vi "ST_parse_results_audit.vi"(7 "data_start_index":i32, 8 "error_in":errorcluster, 11 "results_from_PLC":u8[](array[numeric])) -> (0 "error_out":errorcluster, 3 "results_from_PLC":T1)   [LabVIEW 2020]
uses:
  ST_results_info.ctl
  results_byte_offset/res_REAL_offset.vi
  _misc/byte_array_parser/to_SGL.vi
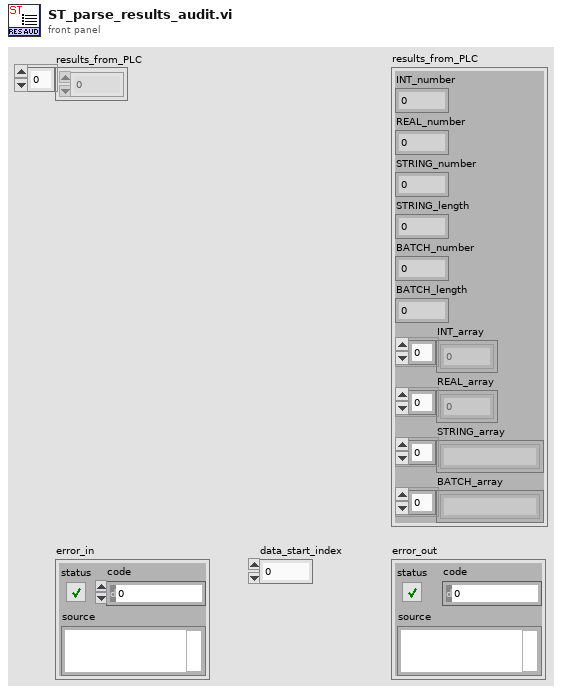
[diagram p1: front panel]
types:
  T1 = typedef "ST_results_info.ctl" = cluster{"INT_number":i32, "REAL_number":i32, "STRING_number":i32, "STRING_length":i32, "BATCH_number":i32, "BATCH_length":i32, "INT_array":i16[], "REAL_array":sgl[], "STRING_array":string[], "BATCH_array":string[]}
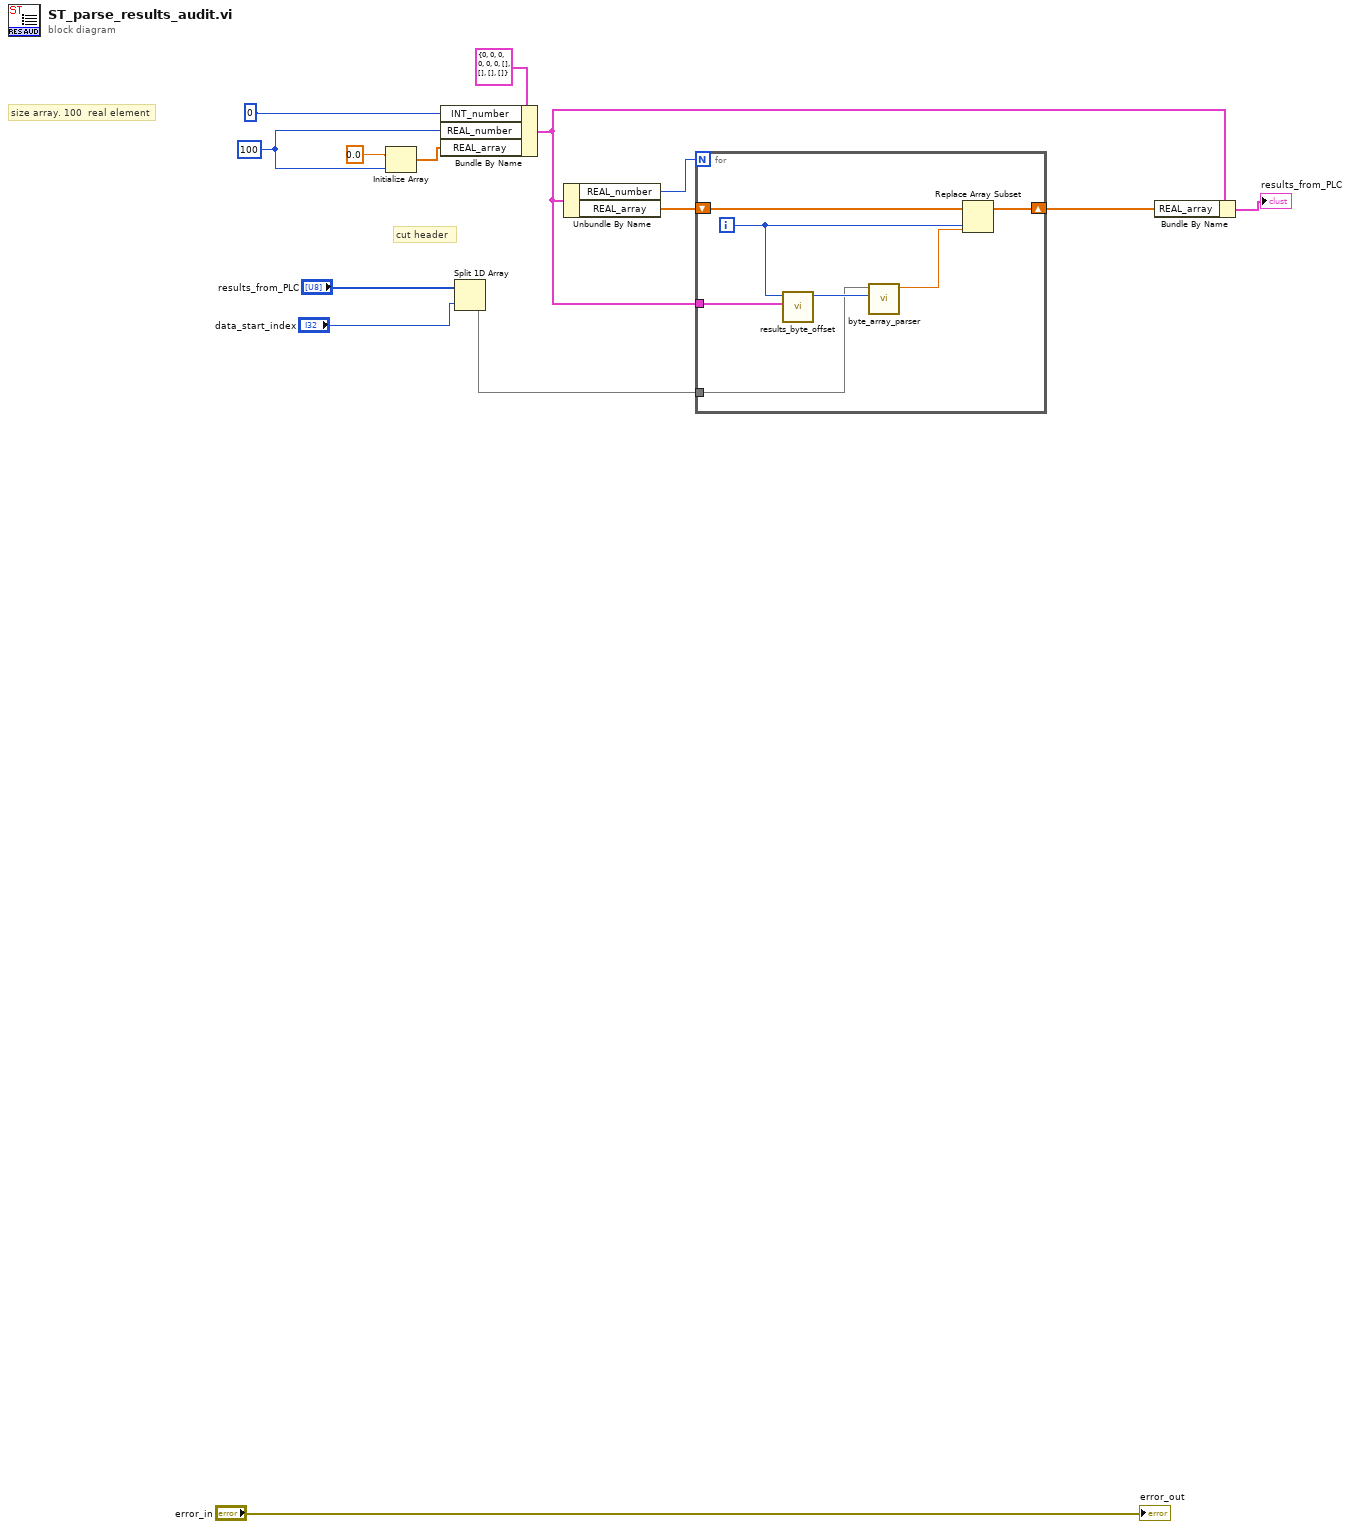
[diagram p0: block diagram]
diagram:
  w10 = 100 ("REAL_number")
  # "size array. 100  real element"
  # "cut header"
  n1 = Initialize Array(sgl 0.0 ("element"), w10) -> (w11:sgl[])
  n2 = Bundle By Name(cluster=T1 {"INT_number"=0, "REAL_number"=0, "STRING_number"=0, "STRING_length"=0, "BATCH_number"=0, "BATCH_length"=0, "INT_array"=[], "REAL_array"=[], "STRING_array"=[], "BATCH_array"=[]} ("ST_reference_info"), "INT_number"=0 ("REAL_number"), "REAL_number"=w10, "REAL_array"=w11) -> (w3:T1)
  n3 = Split 1D Array(array="results_from_PLC", index="data_start_index") -> (second subarray=w1:u8[])  [unwired: 1 out]
  n4 = Unbundle By Name(w3) -> ("REAL_number"=w9:i32, "REAL_array"=w8:sgl[])
  n5 = for {
    N: w9 -> [_]
    shift-right: [w20] -> w5
    shift-left: w8 -> [w21]
    tunnel: w1 -> [w15]
    tunnel: w3 -> [w19]
    i -> [w16]
    n6 = call-poly "results_byte_offset.vi"("ST_results_info"=w19, "REAL_position"=w16) -> ("results_byte_array_offset"=w18:i32)  [unwired: 9 in]
    n7 = call-poly "byte_array_parser.vi"("variable_start_index"=w18, "byte_array"=w15) -> ("SGL"=w17:sgl)  [unwired: 8 in, 1 out]
    n8 = Replace Array Subset(array=w21, new element=w17, index=w16) -> (w20:sgl[])
  }
  n9 = Bundle By Name(cluster=w3, "REAL_array"=w5) -> (→"results_from_PLC":T1)
  "error_out" <- "error_in"
